vi "niRFUtil RFHS Benchmark Simple Profiler.vi"(0 "Reset":bool, 2 "Label":string, 5 "Capture":bool=TRUE, 7 "Error In":errorcluster) -> (4 "Time Profile":cluster{"Time":dbl, "Label":string}[](array[cluster]) {"Time" format="%#.3ps"}, 6 "Total Elapsed Time":dbl format="%#.3ps", 8 "Error Out":errorcluster)   [LabVIEW 2015, in "niRFUtil.lvlib"]
doc: "This is a dead simple easy-to-use Time Profiler. This VI captures the current elapsed time in seconds and saves it together with a label in an array. Drop the Profiler along your error cluster chain to get an aggregated time profile at the end.\n\nThis VI is configured for non-entrant execution which allows to save data between calls in uninitialized shift registers. Don't change this setting! Having the Profiler only one time in memory has some benefits: You can place this profiler multiple times in ANY of your Sub-VIs to capture a profile and collect the results in your very top VI. No need to pass a handle, all times are collected globally without the need for an external global variable.\n\nHOW TO USE\n- Connect the Profiler in any place you'd like to benchmark. You may use the error cluster (errors are ignored and get passed straight through). Optionally pass a string to the \"Label\" terminal to name the current time measurement in the profile. If there's no error wire around, connect any other active wire to a plain structure (e.g. a Flat Sequence) and put the Profiler in there.\n- When done, call the Profiler in your top level VI and pull the results from the \"Time Profile\" terminal. Optionally get the total elapsed time since the last reset from the \"Total Elapsed Time\" terminal.\n- The time reference and the profile are reset automatically on first run. However, you can do it manually by wiring True to the \"Reset\" terminal.\n\nTIME\nThe time marks in the output profile are given in seconds of double precision. Please note that they are not relative to each other, but to a common start reference (i.e. the last reset). The current time is retrieved using LabVIEW's utility \"High Resolution Relative Seconds.vi\".\n\nnick.schwarzenberg@ni.com"
uses:
  niRFUtil.lvlib
panel:
  out "Reference Time":dbl format="%#.3ps"
  # "INPUT"
  # "RESULTS"
  # "REFERENCE"
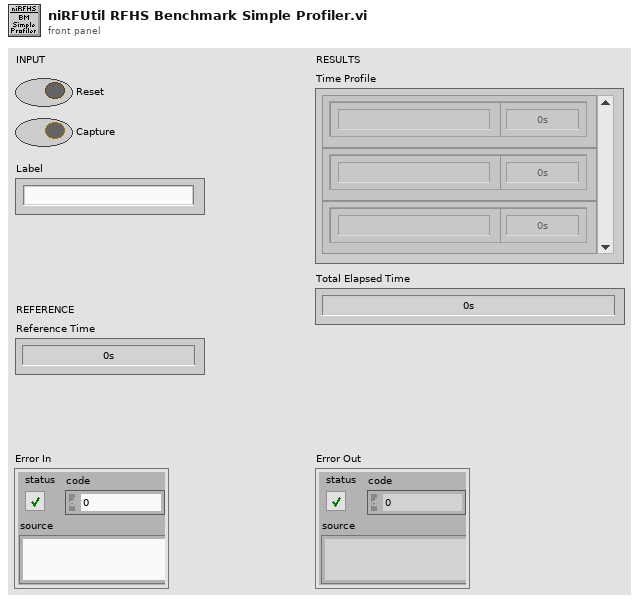
[diagram p1: front panel]
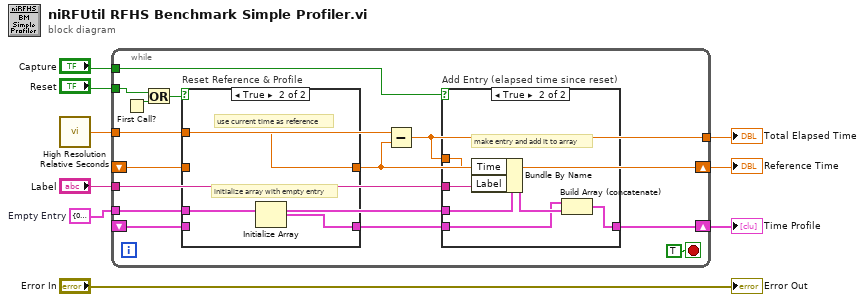
[diagram p0: block diagram]
diagram:
  w3 = cluster{"Time":dbl, "Label":string} {"Time"=0.0, "Label"=""}  # Empty Entry
  n1 = call <vilib>:"High Resolution Relative Seconds.vi"() -> ("relative seconds"=w6:dbl)
  n2 = while {
    tunnel: "Label" -> [w23]
    tunnel: w6 -> [w15]
    tunnel: "Reset" -> [w12]
    shift-right: [w22] -> w7
    shift-left: _ -> [w17]
    tunnel: "Capture" -> [w19]
    tunnel: w3 -> [w14]
    shift-right: [w20] -> w1
    shift-left: _ -> [w18]
    tunnel: [w13] -> w2
    stop <- TRUE stop-if-true
    n3 = First Call?() -> (First Call?: T/F=w10:bool)
    n4 = Or(x=w12, y=w10) -> (x .or. y?=w11:bool)
    n5 = case "Reset Reference & Profile" shown="True" w11 {
      tunnel: [w24 w28] -> w20
      tunnel: w18 -> [w24 _]
      tunnel: w17 -> [w25 _]
      tunnel: [w25 w27] -> w16
      tunnel: w15 -> [_ w28]
      tunnel: w14 -> [_ w26]
      frame False {
      }
      frame True {
        # "use current time as reference"
        # "initialize array with empty entry"
        n6 = Initialize Array(w26) -> (w27:cluster{"Time":dbl, "Label":string}[])  [unwired: 1 in]
      }
    }
    n7 = Subtract(x=w15, y=w20) -> (x-y=w13:dbl)
    n8 = case "Add Entry (elapsed time since reset)" shown="True" w19 {
      tunnel: w23 -> [_ w35]
      tunnel: [w29 w33] -> w22
      tunnel: w14 -> [_ w32]
      tunnel: w13 -> [_ w30]
      tunnel: w16 -> [w29 w31]
      frame False {
      }
      frame True {
        # "make entry and add it to array"
        n9 = Bundle By Name(cluster=w32, "Time"=w30, "Label"=w35) -> (w34:cluster{"Time":dbl, "Label":string})
        n10 = Build Array (concatenate)(w31, w34) -> (w33:cluster{"Time":dbl, "Label":string}[])
      }
    }
  }
  "Time Profile" <- w7
  "Total Elapsed Time" <- w2
  "Reference Time" <- w1
  "Error Out" <- "Error In"
